vi "Create.vi"(8 "error in (no error)":errorcluster, 10 "Owner":refnum<vi>, 11 "Actor in":refnum<class "Actor.lvclass">) -> (0 "error out":errorcluster, 3 "API-Reference":refnum<data-value>)   [LabVIEW 2018, in "Scripting.lvlib" / "Actor.lvclass"]
uses:
  Actor.lvclass
  API-Data.ctl
  Front-Panel State.ctl
  Did Stop.ctl
  All-Enqueuers.ctl
  Broadcast Enqueuers.ctl
  Did Initialize.ctl
  Request-Enqueuers.ctl
  Get State.ctl
  State.ctl
  Stop.ctl
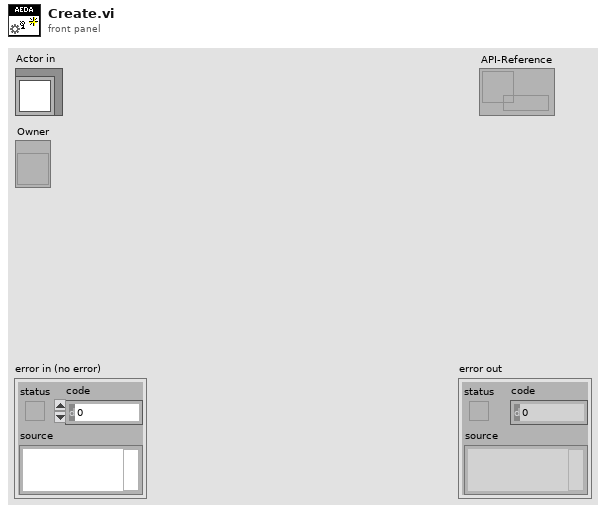
[diagram p1: front panel]
types:
  T1 = typedef "Scripting.lvlib/Actor.lvclass/Front-Panel State.ctl" = enum16{"Don't Show", "Show"}
  T2 = typedef "Scripting.lvlib/Actor.lvclass/All-Enqueuers.ctl" = cluster{"Broadcasts":T3, "Requests":T4}
  T3 = typedef "Scripting.lvlib/Actor.lvclass/Broadcast Enqueuers.ctl" = cluster{"Did Initialize":refnum<user-event>}
  T4 = typedef "Scripting.lvlib/Actor.lvclass/Request-Enqueuers.ctl" = cluster{"Get State":refnum<user-event>, "Stop":refnum<user-event>}
  T5 = typedef "Scripting.lvlib/Actor.lvclass/Did Stop.ctl" = cluster{"State":refnum<class "Actor.lvclass">, "Final Error":errorcluster}
  T6 = typedef "Scripting.lvlib/Actor.lvclass/API-Data.ctl" = cluster{"Launch":refnum<notifier>, "Did Stop Message":refnum<event-registration>, "Did Stop Enqueuer":refnum<user-event>, "Enqueuers":T2}
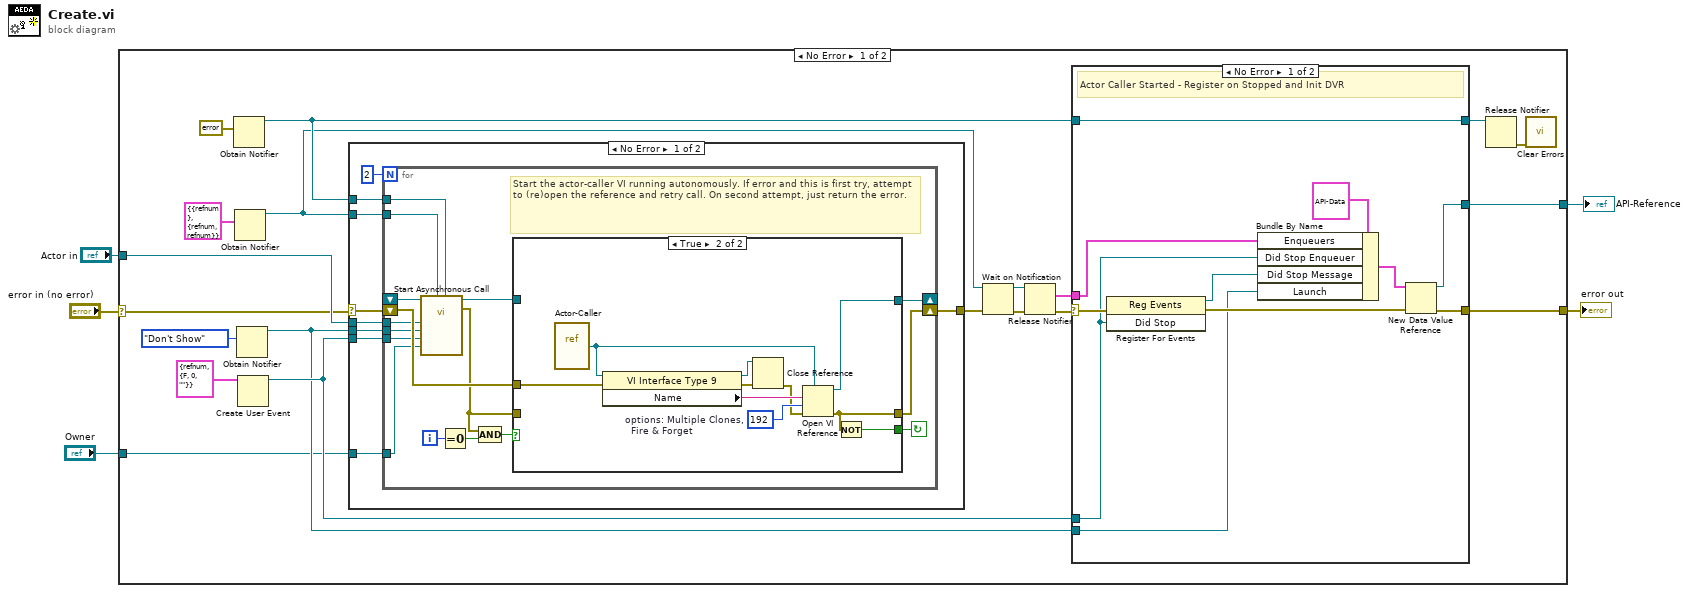
[diagram p0: block diagram]
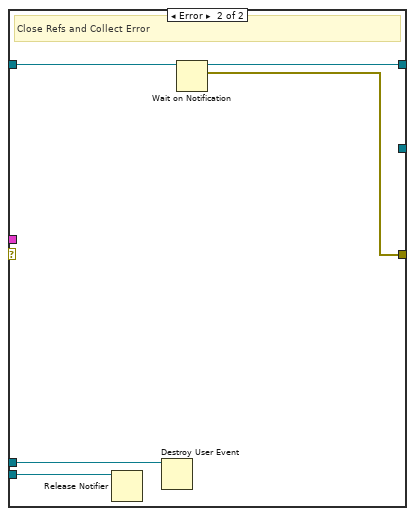
[diagram p4: hidden frame]
diagram:
  n1 = case shown="No Error" "error in (no error)" {
    selector: "error in (no error)" -> [w12 w80]
    tunnel: [w23 w80] -> w4
    tunnel: "Actor in" -> [w20 _]
    tunnel: [w10 _] -> w2
    tunnel: "Owner" -> [w6 _]
    frame No Error {
      n2 = Obtain Notifier(notification data type=errorcluster {"status"=FALSE, "code"=0, "source"=""} ("error constant")) -> (notifier out=w21:refnum<notifier>)  [unwired: 3 in, 2 out]
      n3 = Obtain Notifier(notification data type=T2 {"Broadcasts"={"Did Initialize"=refnum}, "Requests"={"Get State"=refnum, "Stop"=refnum}} ("Actor-Events")) -> (notifier out=w17:refnum<notifier>)  [unwired: 3 in, 2 out]
      n4 = Obtain Notifier(notification data type=Front-Panel_State."Don't Show" ("Front Panel State")) -> (notifier out=w9:refnum<notifier>)  [unwired: 3 in, 2 out]
      n5 = Create User Event(user event datatype=T5 {"State"=refnum, "Final Error"={"status"=FALSE, "code"=0, "source"=""}} ("Did Stop")) -> (user event=w11:refnum<user-event>)  [unwired: 1 in, 1 out]
      n6 = case shown="No Error" w12 {
        selector: w12 -> [w32 w63]
        tunnel: [w33 w63] -> w19
        tunnel: w17 -> [w31 _]
        tunnel: w21 -> [w30 _]
        tunnel: w20 -> [w29 _]
        tunnel: w9 -> [w28 _]
        tunnel: w11 -> [w27 _]
        tunnel: w6 -> [w26 _]
        frame No Error {
          n7 = for {
            N: 2 -> [_]
            shift-right: [w50] -> w33
            shift-left: w32 -> [w45]
            shift-right: [w44] -> _
            shift-left: _ -> [w43]
            tunnel: w31 -> [w37]
            tunnel: w30 -> [w36]
            tunnel: w29 -> [w40]
            tunnel: w28 -> [w39]
            tunnel: w27 -> [w38]
            tunnel: w26 -> [w35]
            i -> [w47]
            stop <- w46 continue-if-true
            # "Start the actor-caller VI running autonomously. If error and this is first try, attempt to (re)open the reference and retry call. On second attempt, just return the error."
            n8 = call-by-ref "Start Asynchronous Call"(reference=w43, "Initialize-Error Passback"=w36, "Enqueuers Passback"=w37, "Owner"=w35, "Did Stop Enqueuer"=w38, "Launch"=w39, "Actor in"=w40) -> (reference out=w42:refnum<vi>, error out=w41:errorcluster)  [unwired: 7 in]
            n9 = Equal To 0?(x=w47) -> (x = 0?=w48:bool)
            n10 = Compound Arithmetic op=AND(w41, w48) -> (w49:bool)
            n11 = case shown="True" w49 {
              tunnel: [w51 w59] -> w44
              tunnel: [w52 w61] -> w50
              tunnel: w41 -> [w52 _]
              tunnel: [_ w62] -> w46
              tunnel: w45 -> [_ w60]
              tunnel: w42 -> [w51 _]
              frame False {
              }
              frame True {
                w57 = 192  # options: Multiple Clones,   Fire & Forget
                n12 = vi-ref "Actor-Caller.vi"() -> (w53:refnum<vi>)
                n13 = property class="VI Interface Type 9"(reference=w53, error in=w60) -> (reference out=w55:refnum<vi>, error out=w56:errorcluster, "Name"=w58:string)
                n14 = Close Reference(reference=w55, error in (no error)=w56) -> (error out=w54:errorcluster)
                n15 = Open VI Reference(type specifier VI Refnum (for type only)=w53, vi path=w58, options=w57, error in (no error)=w54) -> (vi reference=w59:refnum<vi>, error out=w61:errorcluster)  [unwired: 2 in]
                n16 = Not(x=w61) -> (.not. x?=w62:bool)
              }
            }
          }
        }
        frame Error {
        }
      }
      n17 = Wait on Notification(notifier=w17, error in (no error)=w19) -> (notifier out=w16:refnum<notifier>, error out=w15:errorcluster)  [unwired: 2 in, 2 out]
      n18 = Release Notifier(notifier=w16, error in (no error)=w15) -> (last notification=w13:T2, error out=w14:errorcluster)  [unwired: 1 in, 1 out]
      n19 = case shown="No Error" w14 {
        selector: w14 -> [w71 _]
        tunnel: w13 -> [w67 _]
        tunnel: w21 -> [w74 w79]
        tunnel: [w74 w78] -> w24
        tunnel: [w72 w77] -> w23
        tunnel: w11 -> [w64 w76]
        tunnel: w9 -> [w69 w75]
        tunnel: [w66 _] -> w10
        frame No Error {
          # "Actor Caller Started - Register on Stopped and Init DVR"
          n20 = register-events(error in=w71, w64) -> (reference out=w65:refnum<event-registration>, error out=w70:errorcluster)  [unwired: 1 in]
          n21 = Bundle By Name(cluster=T6 {"Launch"=refnum, "Did Stop Message"=refnum, "Did Stop Enqueuer"=refnum, "Enqueuers"={"Broadcasts"={"Did Initialize"=refnum}, "Requests"={"Get State"=refnum, "Stop"=refnum}}} ("API-Data"), "Enqueuers"=w67, "Did Stop Enqueuer"=w64, "Did Stop Message"=w65, "Launch"=w69) -> (w73:T6)
          n22 = New Data Value Reference(data value=w73, error in=w70) -> (data value reference=w66:refnum<data-value>, error out=w72:errorcluster)
        }
        frame Error {
          # "Close Refs and Collect Error"
          n23 = Release Notifier(notifier=w75) -> ()  [unwired: 2 in, 3 out]
          n24 = Destroy User Event(user event=w76) -> ()  [unwired: 1 in, 1 out]
          n25 = Wait on Notification(notifier=w79) -> (notifier out=w78:refnum<notifier>, notification=w77:errorcluster)  [unwired: 3 in, 2 out]
        }
      }
      n26 = Release Notifier(notifier=w24) -> (error out=w7:errorcluster)  [unwired: 2 in, 2 out]
      n27 = call <vilib>:"Clear Errors.vi"("error in (no error)"=w7) -> ()  [unwired: 5 in, 2 out]
    }
    frame Error {
    }
  }
  "error out" <- w4
  "API-Reference" <- w2
